vi "TextControlledInstrumControlToCommands.vi"(9 "Command Array":string[][](array[string]), 10 "Control to Index":T1(c390), 11 "Control in":refnum<vi>) -> (1 "Command Array out":string[][](array[string]), 3 "Control out":refnum<vi>)   [LabVIEW 2021]
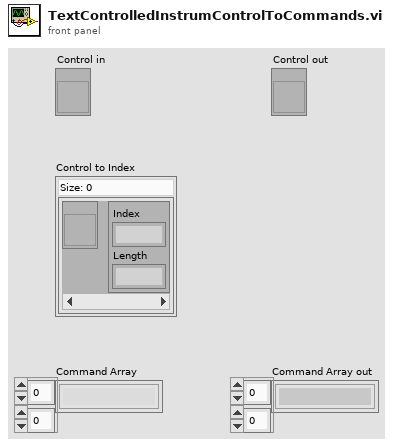
[diagram p1: front panel]
types:
  T1 = map{refnum<vi>, cluster{"Index":i32, "Length":i32}}
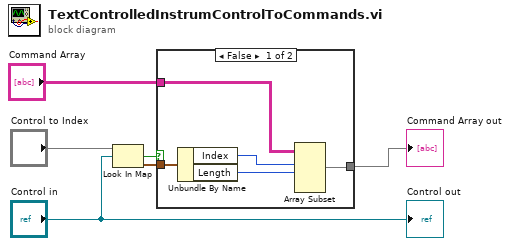
[diagram p0: block diagram]
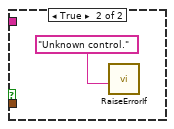
[diagram p2: hidden frame]
diagram:
  n1 = Look In Map(map="Control to Index", key="Control in") -> (key not found?=w4:bool, value=w3:cluster{"Index":i32, "Length":i32})  [unwired: 1 in]
  n2 = case shown="False" w4 {
    tunnel: w3 -> [w11 _]
    tunnel: "Command Array" -> [w8 _]
    tunnel: [w7 _] -> w1
    frame False {
      n3 = Unbundle By Name(w11) -> ("Index"=w10:i32, "Length"=w9:i32)
      n4 = Array Subset(array=w8, index (row)=w10, length (row)=w9) -> (w7:string[][])  [unwired: 2 in]
    }
    frame True {
      n5 = call "RaiseErrorIf.vi"("error message"="Unknown control." ("error source (\" \")")) -> ()  [unwired: 10 in, 1 out]
    }
  }
  "Command Array out" <- w1
  "Control out" <- "Control in"
